vi "Version.vi"(8 "error in (no error)":errorcluster, 11 "lvzstd in":refnum<class "lvzstd.lvclass">) -> (0 "error out":errorcluster, 2 "version":string, 3 "lvzstd out":refnum<class "lvzstd.lvclass">)   [LabVIEW 2020, in "lvzstd.lvlib" / "lvzstd.lvclass"]
uses:
  lvzstd.lvclass
  lvzstd.lvclass/lvzstd.ctl
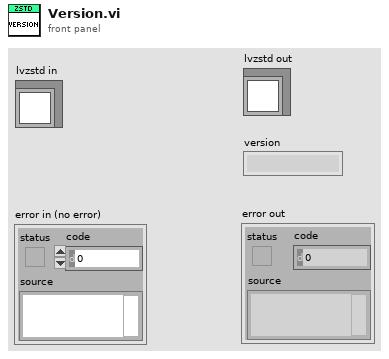
[diagram p1: front panel]
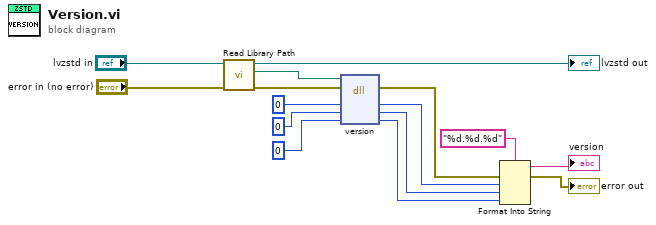
[diagram p0: block diagram]
diagram:
  n1 = call "Read Library Path.vi"("error in (no error)"="error in (no error)", "lvzstd in"="lvzstd in") -> ("error out"=w11:errorcluster, "Library Path"=w13:path, "lvzstd out"=→"lvzstd out":refnum<class "lvzstd.lvclass">)  [unwired: 7 in]
  n2 = dll-call lib="?" fn="version"(path in=w13, error in=w11, "major"=0, "minor"=0 ("major"), "patch"=0 ("major")) -> (error out=w3:errorcluster, "major"=w7:i32, "minor"=w6:i32, "patch"=w5:i32)  [unwired: 2 in, 1 out]
  n3 = Format Into String(format string="%d.%d.%d", error in=w3, w7, w6, w5) -> (resulting string=→"version":string, error out=→"error out":errorcluster)  [unwired: 1 in]
